vi "launcher.vi"   [LabVIEW 2014]
types:
  T1 = enum32{"Invalid", "Standard", "Closed", "Hidden", "Minimized", "Maximized"}
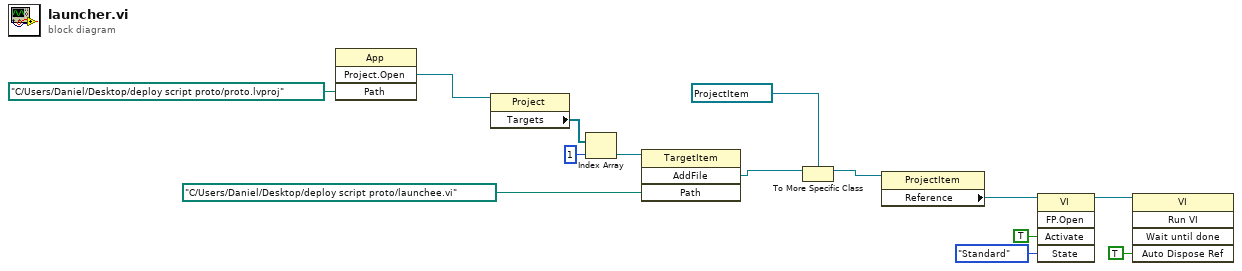
[diagram p0: block diagram]
diagram:
  n1 = invoke class="App" method="Project.Open"("Path"=path "C:/Users/Daniel/Desktop/deploy script proto/proto.lvproj") -> ("Project:Open"=w13:refnum<vi>)  [unwired: 3 in, 3 out]
  n2 = property class="Project"(reference=w13) -> ("Targets"=w12:refnum<vi>[])  [unwired: 1 in, 2 out]
  n3 = Index Array(array=w12, index=1) -> (element=w10:refnum<vi>)
  n4 = invoke class="TargetItem" method="AddFile"(reference=w10, "Path"=path "C:/Users/Daniel/Desktop/deploy script proto/launchee.vi") -> ("AddFile"=w7:refnum<vi>)  [unwired: 2 in, 3 out]
  n5 = To More Specific Class(target class=refnum<vi> refnum ("Add File"), reference=w7) -> (specific class reference=w6:refnum<vi>)  [unwired: 1 in, 1 out]
  n6 = property class="ProjectItem"(reference=w6) -> ("Reference"=w5:refnum<vi>)  [unwired: 1 in, 2 out]
  n7 = invoke class="VI" method="FP.Open"(reference=w5, "Activate"=TRUE ("Activate?"), "State"=T1."Standard") -> (reference out=w4:refnum<vi>)  [unwired: 2 in, 4 out]
  n8 = invoke class="VI" method="Run VI"(reference=w4, "Auto Dispose Ref"=TRUE ("Auto Dispose Reference")) -> ()  [unwired: 3 in, 5 out]
